vi "Pixellate Single.vi"(8 "error in":errorcluster, 10 "Overlay":T1, 11 "BigMAQ in":refnum<class "BigMAQ.lvclass">) -> (0 "error out":errorcluster, 2 "Pixellated Overlay":T1, 3 "BigMAQ out":refnum<class "BigMAQ.lvclass">)   [LabVIEW 2019, in "BigMAQ.lvclass"]
uses:
  BigMAQ.lvclass
  Overlay.ctl
  BigMAQ.lvclass/BigMAQ.ctl
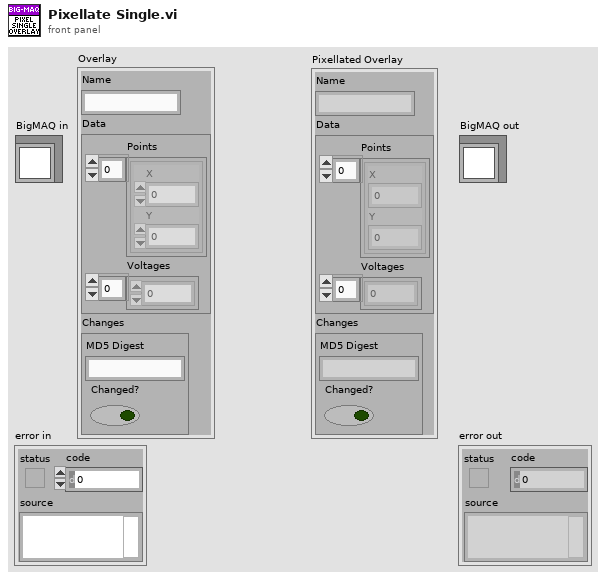
[diagram p1: front panel]
types:
  T1 = typedef "BigMAQ.lvclass/Overlay.ctl" = cluster{"Name":string, "Data":cluster{"Points":cluster{"X":dbl, "Y":dbl}[], "Voltages":dbl[]}, "Changes":cluster{"MD5 Digest":string, "Changed?":bool}}
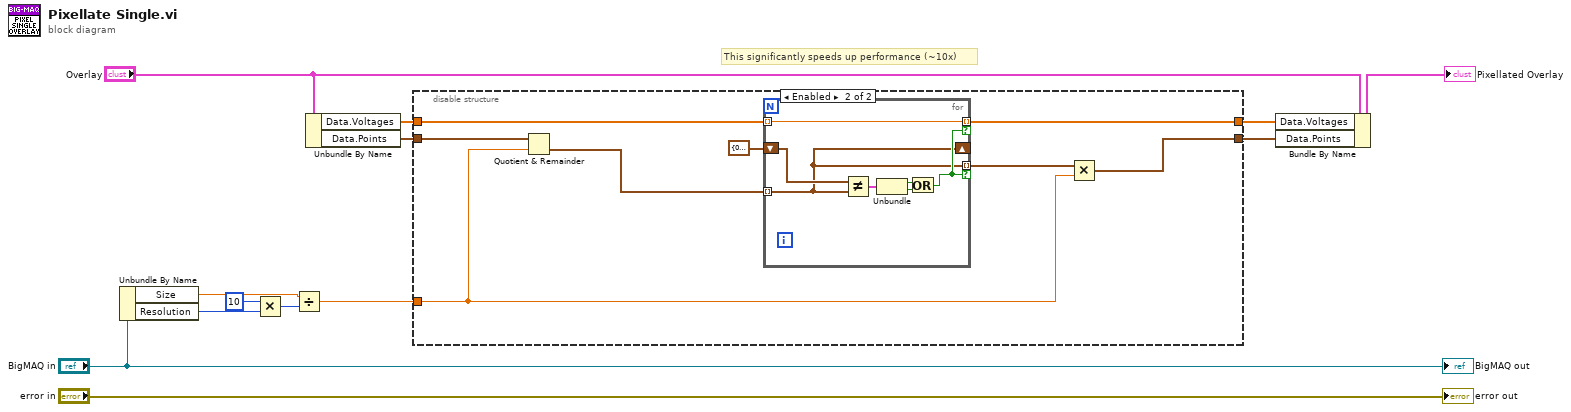
[diagram p0: block diagram]
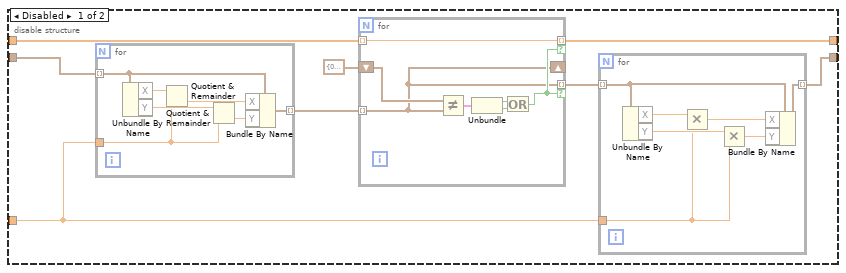
[diagram p2: hidden frame]
diagram:
  # "This significantly speeds up performance (~10x)"
  n1 = Unbundle By Name("BigMAQ in") -> ("Size"=w2:dbl, "Resolution"=w3:i32)
  n2 = Multiply(x=10, y=w3) -> (x*y=w5:i32)
  n3 = Divide(x=w2, y=w5) -> (x/y=w4:dbl)
  n4 = Unbundle By Name("Overlay") -> ("Data.Voltages"=w8:dbl[], "Data.Points"=w12:cluster{"X":dbl, "Y":dbl}[])
  n5 = disable-structure shown="Enabled" {
    disable-tunnel: w12 -> [w21 w47]
    disable-tunnel: [w18 w43] -> w10
    disable-tunnel: [w16 w49] -> w9
    disable-tunnel: w8 -> [w15 w48]
    disable-tunnel: w4 -> [w14 w44]
    frame Disabled {
      n6 = for {
        tunnel: w21 -> [w32] mode=indexing
        tunnel: [w33] -> w19 mode=indexing
        tunnel: w14 -> [w29]
        n7 = Unbundle By Name(w32) -> ("X"=w30:dbl, "Y"=w31:dbl)
        n8 = Quotient & Remainder(x=w30, y=w29) -> (floor(x/y)=w35:dbl)  [unwired: 1 out]
        n9 = Quotient & Remainder(x=w31, y=w29) -> (floor(x/y)=w34:dbl)  [unwired: 1 out]
        n10 = Bundle By Name(cluster=w32, "X"=w35, "Y"=w34) -> (w33:cluster{"X":dbl, "Y":dbl})
      }
      n11 = for {
        shift-right: [w36] -> _
        shift-left: cluster{"X":dbl, "Y":dbl} {"X"=0.0, "Y"=0.0} ("Litho Point") -> [w42]
        tunnel: [w36] -> w17 mode=indexing if=w37
        tunnel: w19 -> [w36] mode=indexing
        tunnel: w15 -> [w38] mode=indexing
        tunnel: [w38] -> w16 mode=indexing if=w37
        n12 = Not Equal?(x=w42, y=w36) -> (x != y?=w41:cluster{"X":bool, "Y":bool})
        n13 = Unbundle(w41) -> ("X"=w40:bool, "Y"=w39:bool)
        n14 = Or(x=w40, y=w39) -> (x .or. y?=w37:bool)
      }
      n15 = for {
        tunnel: [w22] -> w18 mode=indexing
        tunnel: w17 -> [w27] mode=indexing
        tunnel: w14 -> [w23]
        n16 = Unbundle By Name(w27) -> ("X"=w28:dbl, "Y"=w24:dbl)
        n17 = Multiply(x=w28, y=w23) -> (x*y=w26:dbl)
        n18 = Multiply(x=w24, y=w23) -> (x*y=w25:dbl)
        n19 = Bundle By Name(cluster=w27, "X"=w26, "Y"=w25) -> (w22:cluster{"X":dbl, "Y":dbl})
      }
    }
    frame Enabled {
      n20 = Quotient & Remainder(x=w47, y=w44) -> (floor(x/y)=w46:cluster{"X":dbl, "Y":dbl}[])  [unwired: 1 out]
      n21 = for {
        shift-right: [w51] -> _
        shift-left: cluster{"X":dbl, "Y":dbl} {"X"=0.0, "Y"=0.0} ("Litho Point") -> [w57]
        tunnel: [w51] -> w45 mode=indexing if=w52
        tunnel: w46 -> [w51] mode=indexing
        tunnel: w48 -> [w53] mode=indexing
        tunnel: [w53] -> w49 mode=indexing if=w52
        n22 = Not Equal?(x=w57, y=w51) -> (x != y?=w56:cluster{"X":bool, "Y":bool})
        n23 = Unbundle(w56) -> ("X"=w55:bool, "Y"=w54:bool)
        n24 = Or(x=w55, y=w54) -> (x .or. y?=w52:bool)
      }
      n25 = Multiply(x=w45, y=w44) -> (x*y=w43:cluster{"X":dbl, "Y":dbl}[])
    }
  }
  n26 = Bundle By Name(cluster="Overlay", "Data.Voltages"=w9, "Data.Points"=w10) -> (→"Pixellated Overlay":T1)
  "error out" <- "error in"
  "BigMAQ out" <- "BigMAQ in"
